vi "Write Bit.vi"(8 "error in":errorcluster, 9 "To write":bool, 10 "PLC Bit Address":string="B3:0/0", 11 "IP Address:":string="192.168.100.15") -> (0 "error out":errorcluster, 3 "IP Address Out":string="192.168.100.15")   [LabVIEW 2018]
uses:
  <vilib>/ethernetip/ethernetip.lvlib
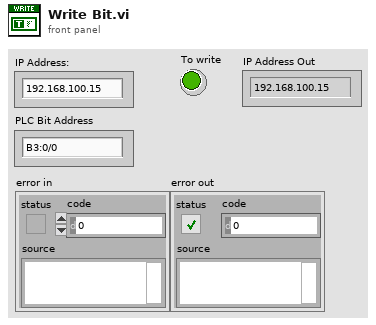
[diagram p1: front panel]
types:
  T1 = typedef "ethernetip.lvlib/ethernetip.ctl" = refnum<k21>
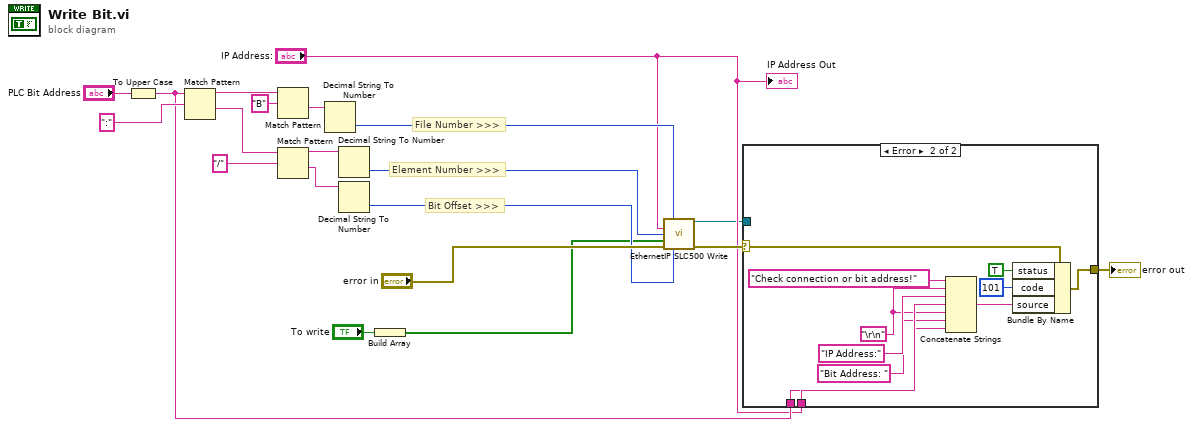
[diagram p0: block diagram]
diagram:
  # "Bit Offset >>>"
  # "Element Number >>>"
  # "File Number >>>"
  n1 = To Upper Case(1:"PLC Bit Address") -> (0:w6:string)
  n2 = Match Pattern(string=w6, regular expression=":") -> (before substring=w19:string, after substring=w14:string)  [unwired: 1 in, 2 out]
  n3 = Match Pattern(string=w19, regular expression="B") -> (after substring=w16:string)  [unwired: 1 in, 3 out]
  n4 = Match Pattern(string=w14, regular expression="/") -> (before substring=w12:string, after substring=w10:string)  [unwired: 1 in, 2 out]
  n5 = Decimal String To Number(string=w16) -> (number=w15:i32)  [unwired: 2 in, 1 out]
  n6 = Decimal String To Number(string=w12) -> (number=w11:i32)  [unwired: 2 in, 1 out]
  n7 = Decimal String To Number(string=w10) -> (number=w4:i32)  [unwired: 2 in, 1 out]
  n8 = Build Array("To write") -> (w2:bool[])
  n9 = call-poly <vilib>:"EthernetIP SLC500 Write.vi"("File Number"=w15, "Network Path"="IP Address:", "Element Number"=w11, "Data"=w2, "error in"="error in", "Bit Offset"=w4) -> ("Session out"=w1:T1, "error out"=w8:errorcluster)  [unwired: 8 in]
  n10 = case shown="Error" w8 {
    selector: w8 -> [w21 w32]
    tunnel: [w21 w31] -> w7
    tunnel: w6 -> [_ w22]
    tunnel: "IP Address:" -> [_ w25]
    tunnel: w1 -> [_ _]
    frame No Error {
    }
    frame Error {
      w24 = "\r\n"
      n11 = Concatenate Strings("Check connection or bit address!" ("source"), w24, "IP Address:", w25, w24, "Bit Address: ", w22) -> (w26:string)
      n12 = Bundle By Name(cluster=w32, "status"=TRUE, "code"=101, "source"=w26) -> (w31:errorcluster)
    }
  }
  "error out" <- w7
  "IP Address Out" <- "IP Address:"
